vi "Print.vi"(8 "error in (no error)":errorcluster, 11 "Message Double in":refnum<class "Message 2D String Array.lvclass">) -> (0 "error out":errorcluster, 2 "String":string, 3 "Message Double out":refnum<class "Message 2D String Array.lvclass">)   [LabVIEW 2016, in "WebSocket Networking.lvlib" / "Message 2D String Array.lvclass"]
doc: "--\nCopyright © 2017 Composed SystemsI All rights reserved.\n\nAuthor: Jon McBee <jon.mcbee@composed.io>\n\nThis library is provided \"AS IS\" ,WITHOUT WARRANTIES OR\nCONDITIONS OF ANY KIND, either express or implied.\n\nComposed Systems -- composed.io\n\nStream 0.0.1.1\nJon McBee - Composed Systems\nCopyright (c) 2017, Composed Systems"
uses:
  <userlib>/Common Components/WebSocket Networking/Message 2D String Array/Message 2D String Array.lvclass
  C:/Program Files (x86)/National Instruments/LabVIEW 2016/user.lib/Composed Systems/Stream/Mediator/Classes/Message Interface/Message Interface.lvclass
  <userlib>/Common Components/WebSocket Networking/Message 2D String Array/Message 2D String Array.lvclass/Message 2D String Array.ctl
  <userlib>/Composed Systems/Stream/Mediator/Classes/Message Interface/Message Interface.lvclass
  <vilib>/addons/_JKI.lib/Serialization/JSON/JKI JSON Serialization.lvlib
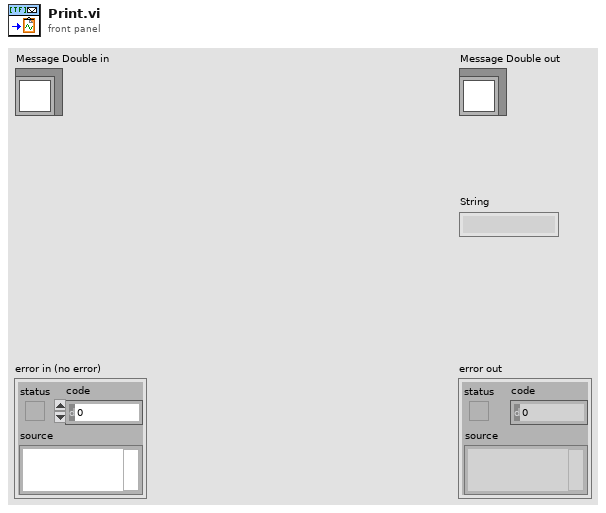
[diagram p1: front panel]
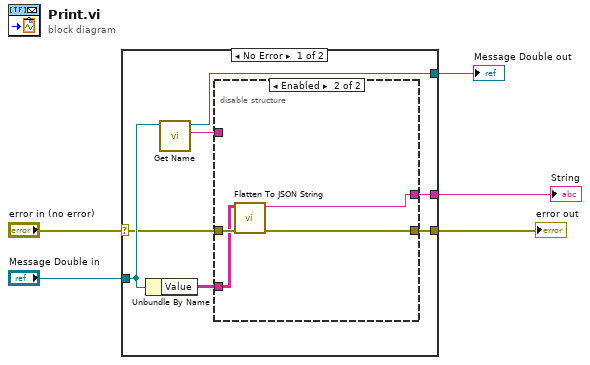
[diagram p0: block diagram]
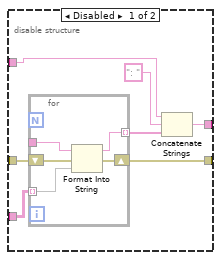
[diagram p2: hidden frame]
diagram:
  n1 = case shown="No Error" "error in (no error)" {
    selector: "error in (no error)" -> [w9 w29]
    tunnel: [w8 w29] -> w4
    tunnel: [w11 w30] -> w2
    tunnel: "Message Double in" -> [w12 w30]
    tunnel: [w6 _] -> w1
    frame No Error {
      n2 = Unbundle By Name(w12) -> ("Value"=w10:string[][])
      n3 = call <userlib>:"Get Name.vi"("Message Interface in"=w12) -> ("Name"=w7:string, "Message Interface out"=w11:refnum<class "Message 2D String Array.lvclass">)  [unwired: 8 in, 1 out]
      n4 = disable-structure shown="Enabled" {
        disable-tunnel: w10 -> [w19 w25]
        disable-tunnel: w9 -> [w18 w28]
        disable-tunnel: [w17 w27] -> w8
        disable-tunnel: w7 -> [w16 _]
        disable-tunnel: [w13 w26] -> w6
        frame Disabled {
          n5 = for {
            tunnel: _ -> [w24]
            tunnel: w19 -> [w23] mode=indexing
            shift-right: [w21] -> w17
            shift-left: w18 -> [w22]
            tunnel: [w20] -> w14 mode=indexing
            n6 = Format Into String(format string=w24, error in=w22, w23) -> (resulting string=w20:string, error out=w21:errorcluster)  [unwired: 1 in]
          }
          n7 = Concatenate Strings(w16, ": ", w14) -> (w13:string)
        }
        frame Enabled {
          n8 = call <vilib>:"Flatten To JSON String.vi"("error in (no error)"=w28, "Variant"=w25) -> ("error out"=w27:errorcluster, "JSON String"=w26:string)  [unwired: 8 in]
        }
      }
    }
    frame Error {
    }
  }
  "error out" <- w4
  "Message Double out" <- w2
  "String" <- w1
